vi "Write Sub Panel Prod.vi"(8 "error in (no error)":errorcluster, 10 "Sub Panel Prod":refnum<vi>, 11 "Bakery Actor in":refnum<class "Bakery Actor.lvclass">) -> (0 "error out":errorcluster, 3 "Bakery Actor out":refnum<class "Bakery Actor.lvclass">)   [LabVIEW 2019, in "Bakery Actor.lvlib" / "Bakery Actor.lvclass"]
uses:
  Bakery Actor.lvclass
  Bakery Actor.lvclass/Bakery Actor.ctl
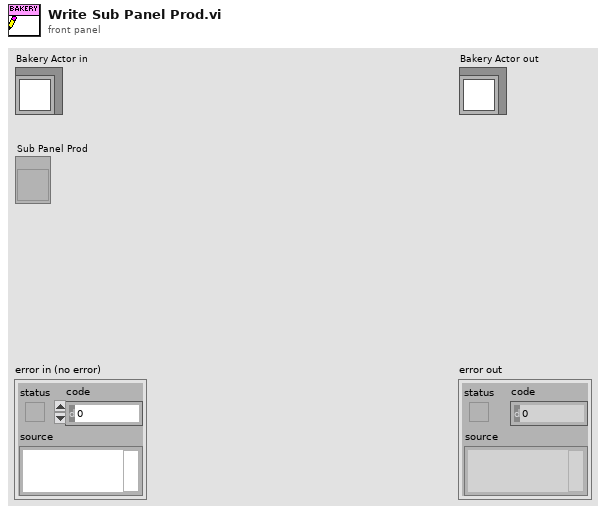
[diagram p1: front panel]
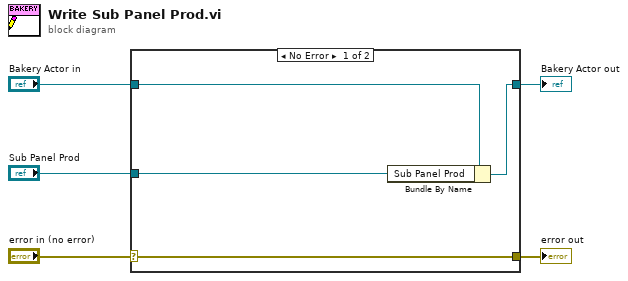
[diagram p0: block diagram]
diagram:
  n1 = case shown="No Error" "error in (no error)" {
    selector: "error in (no error)" -> [w9 w10]
    tunnel: [w9 w10] -> w4
    tunnel: [w7 w11] -> w2
    tunnel: "Bakery Actor in" -> [w8 w11]
    tunnel: "Sub Panel Prod" -> [w6 _]
    frame No Error {
      n2 = Bundle By Name(cluster=w8, "Sub Panel Prod"=w6) -> (w7:refnum<class "Bakery Actor.lvclass">)
    }
    frame Error {
    }
  }
  "error out" <- w4
  "Bakery Actor out" <- w2
